vi "Expand Pathroot.vi"(7 "Application Directory (Default)":path, 10 "Path":path) -> (2 "Path out":path)   [LabVIEW 2011, in "VITesterUtilities.lvlib"]
uses:
  Libraries/VITesterUtilities.lvlib
  <userlib>/_OpenG.lib/file/file.llb/Valid Path - Traditional__ogtk.vi
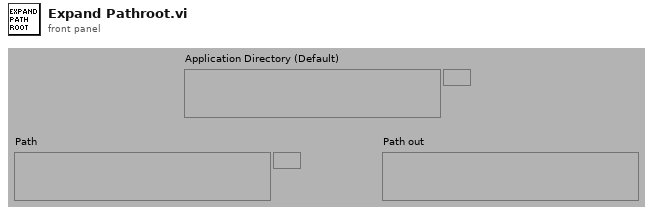
[diagram p1: front panel]
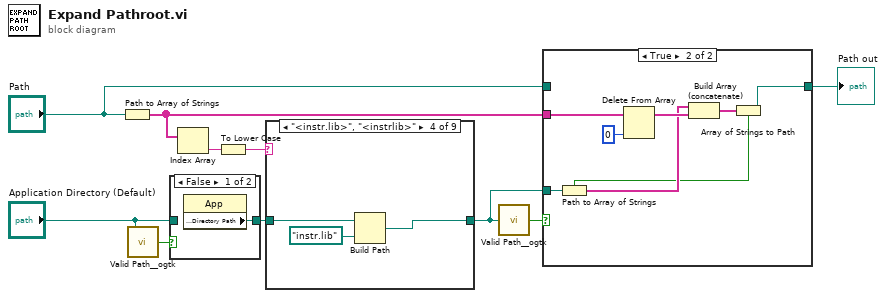
[diagram p0: block diagram]
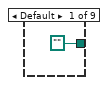
[diagram p4: hidden frame]
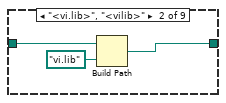
[diagram p5: hidden frame]
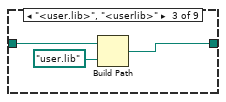
[diagram p6: hidden frame]
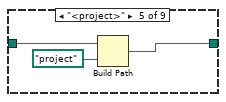
[diagram p7: hidden frame]
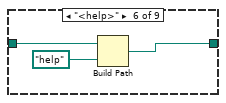
[diagram p8: hidden frame]
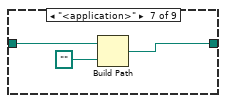
[diagram p9: hidden frame]
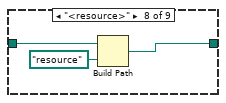
[diagram p10: hidden frame]
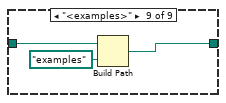
[diagram p11: hidden frame]
diagram:
  n1 = Path to Array of Strings(0:"Path") -> (2:w4:string[])  [unwired: 1 out]
  n2 = call-poly <userlib>:"Valid Path__ogtk.vi"("path"="Application Directory (Default)") -> ("valid"=w7:bool)
  n3 = case shown="False" w7 {
    tunnel: [w11 w12] -> w8
    tunnel: "Application Directory (Default)" -> [_ w12]
    frame False {
      n4 = property class="App"() -> ("Application:Directory Path"=w11:path)  [unwired: 2 in, 2 out]
    }
    frame True {
    }
  }
  n5 = Index Array(array=w4) -> (element=w10:string)  [unwired: 1 in]
  n6 = To Lower Case(string=w10) -> (all lower case string=w9:string)
  n7 = case shown="\"<instr.lib>\", \"<instrlib>\"" w9 {
    tunnel: w8 -> [_ w16 w19 w22 w25 w28 w31 w34 w37]
    tunnel: [path "" w14 w17 w20 w23 w26 w29 w32 w35] -> w3
    frame Default {
    }
    frame "<vi.lib>", "<vilib>" {
      n8 = Build Path(base path=w16, name or relative path=path "vi.lib") -> (appended path=w14:path)
    }
    frame "<user.lib>", "<userlib>" {
      n9 = Build Path(base path=w19, name or relative path=path "user.lib") -> (appended path=w17:path)
    }
    frame "<instr.lib>", "<instrlib>" {
      n10 = Build Path(base path=w22, name or relative path=path "instr.lib") -> (appended path=w20:path)
    }
    frame "<project>" {
      n11 = Build Path(base path=w25, name or relative path=path "project") -> (appended path=w23:path)
    }
    frame "<help>" {
      n12 = Build Path(base path=w28, name or relative path=path "help") -> (appended path=w26:path)
    }
    frame "<application>" {
      n13 = Build Path(base path=w31, name or relative path=path "") -> (appended path=w29:path)
    }
    frame "<resource>" {
      n14 = Build Path(base path=w34, name or relative path=path "resource") -> (appended path=w32:path)
    }
    frame "<examples>" {
      n15 = Build Path(base path=w37, name or relative path=path "examples") -> (appended path=w35:path)
    }
  }
  n16 = call-poly <userlib>:"Valid Path__ogtk.vi"("path"=w3) -> ("valid"=w5:bool)
  n17 = case shown="True" w5 {
    tunnel: w4 -> [_ w45]
    tunnel: w3 -> [_ w46]
    tunnel: "Path" -> [w38 _]
    tunnel: [w38 w39] -> w1
    frame False {
    }
    frame True {
      n18 = Path to Array of Strings(0:w46) -> (1:w40:bool, 2:w42:string[])
      n19 = Delete From Array(array=w45, index=0) -> (array with subset deleted=w43:string[])  [unwired: 1 in, 1 out]
      n20 = Build Array (concatenate)(w42, w43) -> (w41:string[])
      n21 = Array of Strings to Path(0:w41, 1:w40) -> (2:w39:path)
    }
  }
  "Path out" <- w1
